vi "Read.vi"(7 "length":u16, 8 "error in (no error)":errorcluster, 9 "Start address":string, 10 "Read Type":variant, 11 "MelsecTCP in":refnum<class "MelsecFxLinks.lvclass">) -> (0 "error out":errorcluster, 2 "Data":variant, 3 "MelsecTCP out":refnum<class "MelsecFxLinks.lvclass">)   [LabVIEW 2020, in "MelsecFxLinks.lvclass"]
uses:
  MelsecFxLinks.lvclass
  C:/Users/Fred Guo/Desktop/API_Salcomp_CMES/Libraries/HslCommunication/HslCommunication.dll
  HslCommunication.dll
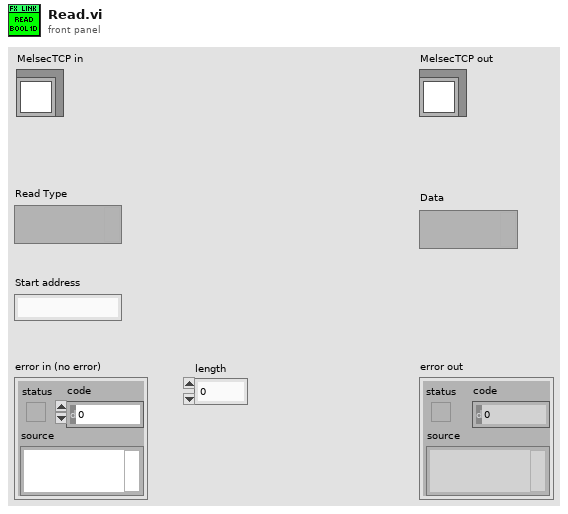
[diagram p1: front panel]
types:
  T1 = typedef "Type Descriptor Enumeration__ogtk.ctl" = enum8{"<Null>", "I8", "I16", "I32", "I64", "U8", "U16", "U32", "U64", "SGL", "DBL", "EXT", "CSG", "CDB", "CXT", "0x0F", "0x10", "0x11", "0x12", "0x13", "0x14", "Enum U8", "Enum U16", "Enum U32", "Enum U64", "SGL PQ", "DBL PQ", "EXT PQ", "CSG PQ", "CDB PQ", "CXT PQ", "0x1F", "0x20", "Boolean", "0x22", "0x23", "0x24", "0x25", "0x26", "0x27", "0x28", "0x29", "0x2A", "0x2B", "0x2C", "0x2D", "0x2E", "0x2F", "String", "0x31", "Path", "Pict", "0x34", "0x35", "0x36", "DAQ", "0x38", "0x39", "0x3A", "0x3B", "0x3C", "0x3D", "0x3E", "0x3F", "Array", "0x41", "0x42", "0x43", "0x44", "0x45", "0x46", "0x47", "0x48", "0x49", "0x4A", "0x4B", "0x4C", "0x4D", "0x4E", "0x4F", "Cluster", "0x51", "0x52", "Variant", "Waveform", "0x55", "0x56", "0x57", "0x58", "0x59", "0x5A", "0x5B", "0x5C", "0x5D", "0x5E", "Fixed Point", "0x60", "0x61", "0x62", "0x63", "0x64", "0x65", "0x66", "0x67", "0x68", "0x69", "0x6A", "0x6B", "0x6C", "0x6D", "0x6E", "0x6F", "Refnum", "0x71", "0x72", "Set Collection", "Map Collection"}
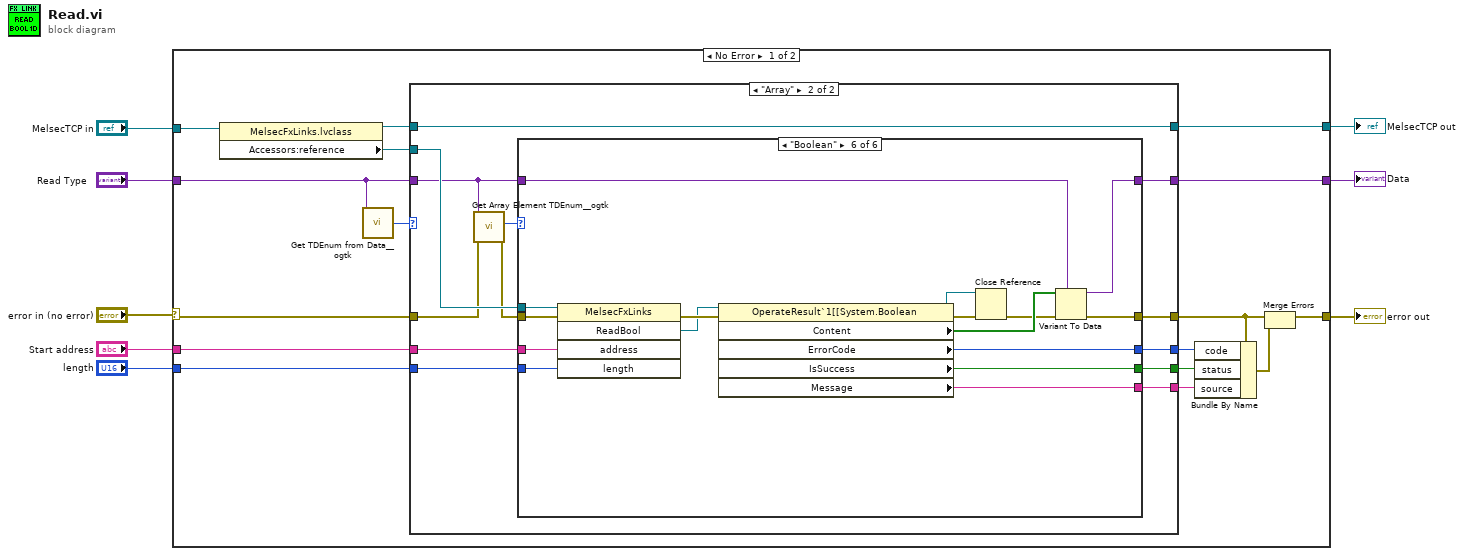
[diagram p0: block diagram]
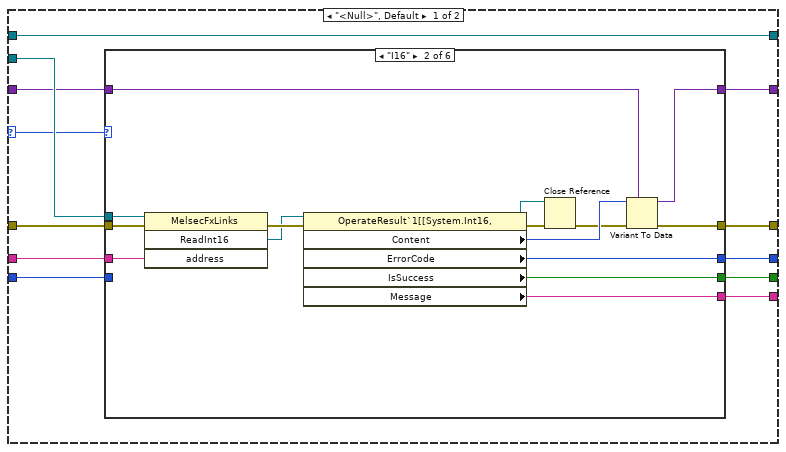
[diagram p2: hidden frame]
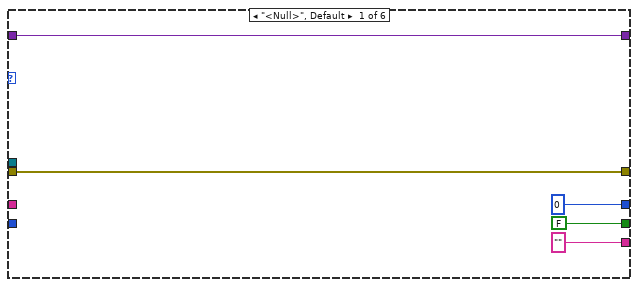
[diagram p3: hidden frame]
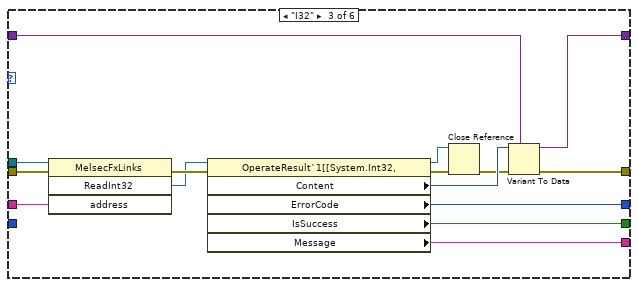
[diagram p4: hidden frame]
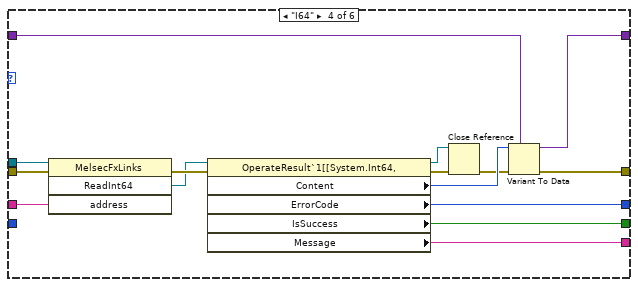
[diagram p5: hidden frame]
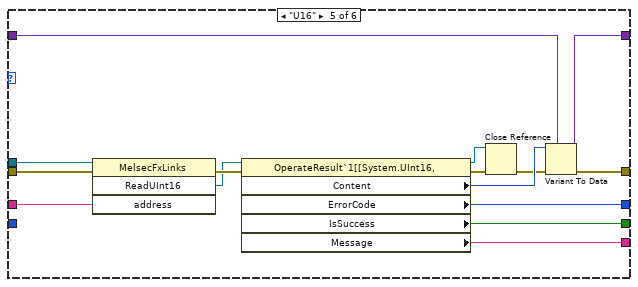
[diagram p6: hidden frame]
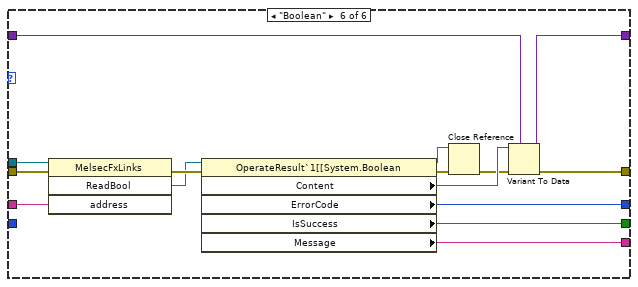
[diagram p7: hidden frame]
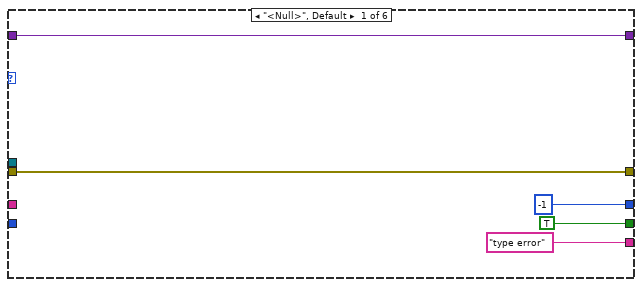
[diagram p8: hidden frame]
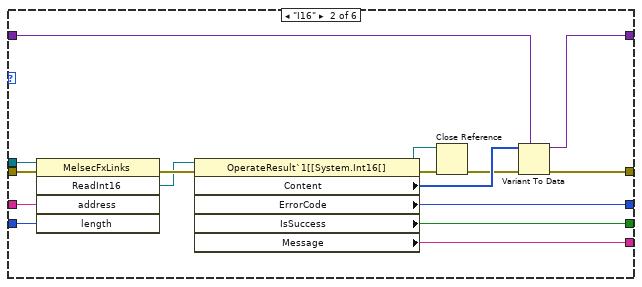
[diagram p9: hidden frame]
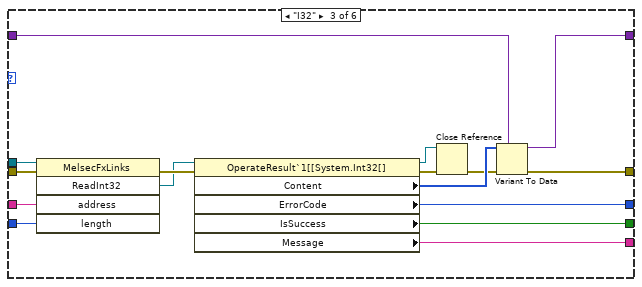
[diagram p10: hidden frame]
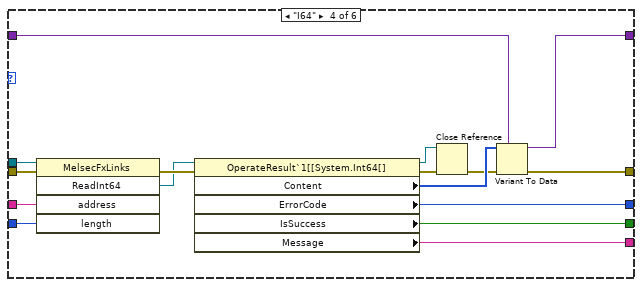
[diagram p11: hidden frame]
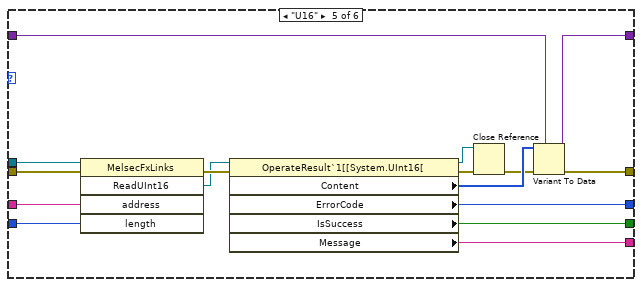
[diagram p12: hidden frame]
diagram:
  n1 = case shown="No Error" "error in (no error)" {
    selector: "error in (no error)" -> [w20 w217]
    tunnel: "MelsecTCP in" -> [w24 w216]
    tunnel: [w9 w216] -> w8
    tunnel: "Start address" -> [w22 _]
    tunnel: [w16 w217] -> w2
    tunnel: [w19 w215] -> w6
    tunnel: "length" -> [w21 _]
    tunnel: "Read Type" -> [w18 w215]
    frame No Error {
      n2 = property class="MelsecFxLinks.lvclass"(reference=w24) -> (reference out=w10:refnum<class "MelsecFxLinks.lvclass">, "Accessors:reference"=w23:refnum<k24>)  [unwired: 1 in, 1 out]
      n3 = call <userlib>:"Get TDEnum from Data__ogtk.vi"("Data"=w18) -> ("Type Descriptor Enumeration"=w17:T1)  [unwired: 4 in]
      n4 = case shown="\"Array\"" w17 {
        selector: w17 -> [w29 _]
        tunnel: w23 -> [w36 w129]
        tunnel: w22 -> [w35 w128]
        tunnel: w21 -> [w34 w127]
        tunnel: w20 -> [w30 w122]
        tunnel: [w33 w126] -> w19
        tunnel: [w32 w125] -> w12
        tunnel: w18 -> [w31 w124]
        tunnel: [w28 w120] -> w15
        tunnel: [w26 w118] -> w13
        tunnel: [w27 w119] -> w14
        tunnel: [w25 w117] -> w9
        tunnel: w10 -> [w25 w117]
        frame "<Null>", Default {
          n5 = case shown="\"I16\"" w29 {
            tunnel: w36 -> [_ w56 w71 w86 w101 w102]
            tunnel: w35 -> [_ w55 w70 w85 w100 w116]
            tunnel: w34 -> [_ _ _ _ _ _]
            tunnel: w30 -> [w41 w54 w69 w84 w99 w115]
            tunnel: [w41 w47 w62 w77 w92 w108] -> w32
            tunnel: [w37 w46 w61 w76 w91 w107] -> w33
            tunnel: [0 ("ErrorCode") w45 w60 w75 w90 w106] -> w28
            tunnel: [FALSE ("IsSuccess") w44 w59 w74 w89 w105] -> w27
            tunnel: ["" ("Message") w43 w58 w73 w88 w104] -> w26
            tunnel: w31 -> [w37 w42 w57 w72 w87 w103]
            frame "<Null>", Default {
            }
            frame "I16" {
              n6 = invoke class="MelsecFxLinks" method="ReadInt16"(reference=w56, error in=w54, "address"=w55) -> (error out=w53:errorcluster, "ReadInt16"=w51:refnum<k24>)  [unwired: 1 in, 2 out]
              n7 = property class="OperateResult`1[[System.Int16, "(reference=w51, error in=w53) -> (reference out=w50:refnum<k24>, error out=w52:errorcluster, "Content"=w49:i16, "ErrorCode"=w45:i32, "IsSuccess"=w44:bool, "Message"=w43:string)
              n8 = Close Reference(reference=w50, error in (no error)=w52) -> (error out=w48:errorcluster)
              n9 = Variant To Data(error in=w48, type=w42, Variant=w49) -> (data=w46:variant, error out=w47:errorcluster)
            }
            frame "I32" {
              n10 = invoke class="MelsecFxLinks" method="ReadInt32"(reference=w71, error in=w69, "address"=w70) -> (error out=w68:errorcluster, "ReadInt32"=w66:refnum<k24>)  [unwired: 1 in, 2 out]
              n11 = property class="OperateResult`1[[System.Int32, "(reference=w66, error in=w68) -> (reference out=w65:refnum<k24>, error out=w67:errorcluster, "Content"=w64:i32, "ErrorCode"=w60:i32, "IsSuccess"=w59:bool, "Message"=w58:string)
              n12 = Close Reference(reference=w65, error in (no error)=w67) -> (error out=w63:errorcluster)
              n13 = Variant To Data(error in=w63, type=w57, Variant=w64) -> (data=w61:variant, error out=w62:errorcluster)
            }
            frame "I64" {
              n14 = invoke class="MelsecFxLinks" method="ReadInt64"(reference=w86, error in=w84, "address"=w85) -> (error out=w83:errorcluster, "ReadInt64"=w81:refnum<k24>)  [unwired: 1 in, 2 out]
              n15 = property class="OperateResult`1[[System.Int64, "(reference=w81, error in=w83) -> (reference out=w80:refnum<k24>, error out=w82:errorcluster, "Content"=w79:i64, "ErrorCode"=w75:i32, "IsSuccess"=w74:bool, "Message"=w73:string)
              n16 = Close Reference(reference=w80, error in (no error)=w82) -> (error out=w78:errorcluster)
              n17 = Variant To Data(error in=w78, type=w72, Variant=w79) -> (data=w76:variant, error out=w77:errorcluster)
            }
            frame "U16" {
              n18 = invoke class="MelsecFxLinks" method="ReadUInt16"(reference=w101, error in=w99, "address"=w100) -> (error out=w98:errorcluster, "ReadUInt16"=w96:refnum<k24>)  [unwired: 1 in, 2 out]
              n19 = property class="OperateResult`1[[System.UInt16,"(reference=w96, error in=w98) -> (reference out=w95:refnum<k24>, error out=w97:errorcluster, "Content"=w94:u16, "ErrorCode"=w90:i32, "IsSuccess"=w89:bool, "Message"=w88:string)
              n20 = Close Reference(reference=w95, error in (no error)=w97) -> (error out=w93:errorcluster)
              n21 = Variant To Data(error in=w93, type=w87, Variant=w94) -> (data=w91:variant, error out=w92:errorcluster)
            }
            frame "Boolean" {
              n22 = invoke class="MelsecFxLinks" method="ReadBool"(reference=w102, error in=w115, "address"=w116) -> (error out=w114:errorcluster, "ReadBool"=w112:refnum<k24>)  [unwired: 1 in, 2 out]
              n23 = property class="OperateResult`1[[System.Boolean"(reference=w112, error in=w114) -> (reference out=w111:refnum<k24>, error out=w113:errorcluster, "Content"=w110:bool, "ErrorCode"=w106:i32, "IsSuccess"=w105:bool, "Message"=w104:string)
              n24 = Close Reference(reference=w111, error in (no error)=w113) -> (error out=w109:errorcluster)
              n25 = Variant To Data(error in=w109, type=w103, Variant=w110) -> (data=w107:variant, error out=w108:errorcluster)
            }
          }
        }
        frame "Array" {
          n26 = call <userlib>:"Get Array Element TDEnum__ogtk.vi"("error in (no error)"=w122, "Array"=w124) -> ("error out"=w121:errorcluster, "Element Type"=w123:T1)  [unwired: 8 in]
          n27 = case shown="\"Boolean\"" w123 {
            tunnel: w129 -> [_ w150 w166 w182 w198 w199]
            tunnel: w128 -> [_ w149 w165 w181 w197 w214]
            tunnel: w127 -> [_ w148 w164 w180 w196 w213]
            tunnel: w121 -> [w134 w147 w163 w179 w195 w212]
            tunnel: [w134 w140 w156 w172 w188 w205] -> w125
            tunnel: [w130 w139 w155 w171 w187 w204] -> w126
            tunnel: [-1 ("ErrorCode") w138 w154 w170 w186 w203] -> w120
            tunnel: [TRUE ("IsSuccess") w137 w153 w169 w185 w202] -> w119
            tunnel: ["type error" ("Message") w136 w152 w168 w184 w201] -> w118
            tunnel: w124 -> [w130 w135 w151 w167 w183 w200]
            frame "<Null>", Default {
            }
            frame "I16" {
              n28 = invoke class="MelsecFxLinks" method="ReadInt16"(reference=w150, error in=w147, "address"=w149, "length"=w148) -> (error out=w146:errorcluster, "ReadInt16"=w144:refnum<k24>)  [unwired: 1 in, 3 out]
              n29 = property class="OperateResult`1[[System.Int16[]"(reference=w144, error in=w146) -> (reference out=w143:refnum<k24>, error out=w145:errorcluster, "Content"=w142:i16[], "ErrorCode"=w138:i32, "IsSuccess"=w137:bool, "Message"=w136:string)
              n30 = Close Reference(reference=w143, error in (no error)=w145) -> (error out=w141:errorcluster)
              n31 = Variant To Data(error in=w141, type=w135, Variant=w142) -> (data=w139:variant, error out=w140:errorcluster)
            }
            frame "I32" {
              n32 = invoke class="MelsecFxLinks" method="ReadInt32"(reference=w166, error in=w163, "address"=w165, "length"=w164) -> (error out=w162:errorcluster, "ReadInt32"=w160:refnum<k24>)  [unwired: 1 in, 3 out]
              n33 = property class="OperateResult`1[[System.Int32[]"(reference=w160, error in=w162) -> (reference out=w159:refnum<k24>, error out=w161:errorcluster, "Content"=w158:i32[], "ErrorCode"=w154:i32, "IsSuccess"=w153:bool, "Message"=w152:string)
              n34 = Close Reference(reference=w159, error in (no error)=w161) -> (error out=w157:errorcluster)
              n35 = Variant To Data(error in=w157, type=w151, Variant=w158) -> (data=w155:variant, error out=w156:errorcluster)
            }
            frame "I64" {
              n36 = invoke class="MelsecFxLinks" method="ReadInt64"(reference=w182, error in=w179, "address"=w181, "length"=w180) -> (error out=w178:errorcluster, "ReadInt64"=w176:refnum<k24>)  [unwired: 1 in, 3 out]
              n37 = property class="OperateResult`1[[System.Int64[]"(reference=w176, error in=w178) -> (reference out=w175:refnum<k24>, error out=w177:errorcluster, "Content"=w174:i64[], "ErrorCode"=w170:i32, "IsSuccess"=w169:bool, "Message"=w168:string)
              n38 = Close Reference(reference=w175, error in (no error)=w177) -> (error out=w173:errorcluster)
              n39 = Variant To Data(error in=w173, type=w167, Variant=w174) -> (data=w171:variant, error out=w172:errorcluster)
            }
            frame "U16" {
              n40 = invoke class="MelsecFxLinks" method="ReadUInt16"(reference=w198, error in=w195, "address"=w197, "length"=w196) -> (error out=w194:errorcluster, "ReadUInt16"=w192:refnum<k24>)  [unwired: 1 in, 3 out]
              n41 = property class="OperateResult`1[[System.UInt16["(reference=w192, error in=w194) -> (reference out=w191:refnum<k24>, error out=w193:errorcluster, "Content"=w190:u16[], "ErrorCode"=w186:i32, "IsSuccess"=w185:bool, "Message"=w184:string)
              n42 = Close Reference(reference=w191, error in (no error)=w193) -> (error out=w189:errorcluster)
              n43 = Variant To Data(error in=w189, type=w183, Variant=w190) -> (data=w187:variant, error out=w188:errorcluster)
            }
            frame "Boolean" {
              n44 = invoke class="MelsecFxLinks" method="ReadBool"(reference=w199, error in=w212, "address"=w214, "length"=w213) -> (error out=w211:errorcluster, "ReadBool"=w209:refnum<k24>)  [unwired: 1 in, 3 out]
              n45 = property class="OperateResult`1[[System.Boolean"(reference=w209, error in=w211) -> (reference out=w208:refnum<k24>, error out=w210:errorcluster, "Content"=w207:bool[], "ErrorCode"=w203:i32, "IsSuccess"=w202:bool, "Message"=w201:string)
              n46 = Close Reference(reference=w208, error in (no error)=w210) -> (error out=w206:errorcluster)
              n47 = Variant To Data(error in=w206, type=w200, Variant=w207) -> (data=w204:variant, error out=w205:errorcluster)
            }
          }
        }
      }
      n48 = Bundle By Name(cluster=w12, "code"=w15, "status"=w14, "source"=w13) -> (w11:errorcluster)
      n49 = Merge Errors(w12, w11) -> (w16:errorcluster)
    }
    frame Error {
    }
  }
  "error out" <- w2
  "MelsecTCP out" <- w8
  "Data" <- w6
